vi "make_exp_graph.vi"(8 "Offset":dbl, 9 "Damping":dbl, 10 "Amplitude":dbl, 11 "Tau Array In":dbl[](array[numeric])) -> (0 "Offset Out":dbl, 1 "Damping Out":dbl, 2 "Amplitude Out":dbl, 3 "output cluster":cluster{dbl[], dbl[]})   [LabVIEW 2015]
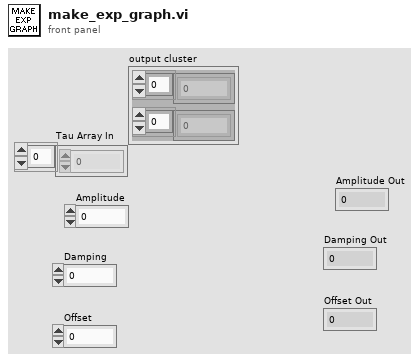
[diagram p1: front panel]
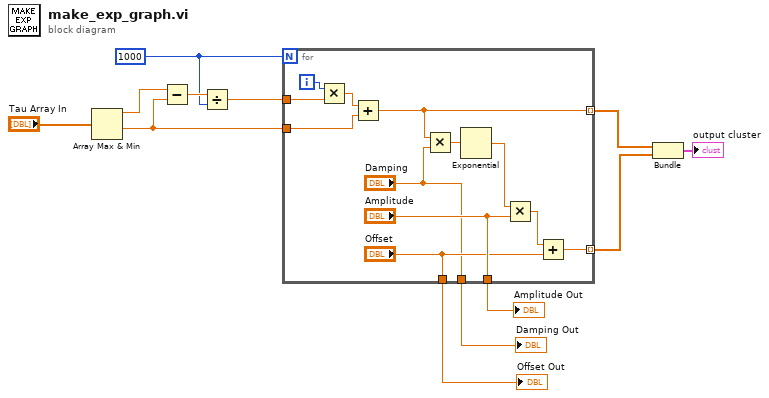
[diagram p0: block diagram]
diagram:
  w9 = 1000
  n1 = Array Max & Min(array="Tau Array In") -> (max value=w11:dbl, min value=w7:dbl)  [unwired: 2 out]
  n2 = Subtract(x=w11, y=w7) -> (x-y=w10:dbl)
  n3 = Divide(x=w10, y=w9) -> (x/y=w8:dbl)
  n4 = for {
    N: w9 -> [_]
    tunnel: w8 -> [w23]
    tunnel: w7 -> [w21]
    tunnel: [w16] -> w3 mode=indexing
    tunnel: [w19] -> w2 mode=indexing
    tunnel: ["Amplitude"] -> w6
    tunnel: ["Damping"] -> w5
    tunnel: ["Offset"] -> w4
    i -> [w24]
    n5 = Multiply(x=w24, y=w23) -> (x*y=w22:dbl)
    n6 = Add(x=w22, y=w21) -> (x+y=w16:dbl)
    n7 = Multiply(x=w16, y="Damping") -> (x*y=w14:dbl)
    n8 = Exponential(1:w14) -> (0:w13:dbl)
    n9 = Multiply(x=w13, y="Amplitude") -> (x*y=w20:dbl)
    n10 = Add(x=w20, y="Offset") -> (x+y=w19:dbl)
  }
  "Amplitude Out" <- w6
  "Damping Out" <- w5
  "Offset Out" <- w4
  n11 = Bundle(w3, w2) -> (→"output cluster":cluster{dbl[], dbl[]})  [unwired: 1 in]
